vi "Terminal-Core-InitializeNotifiers.vi"(0 "comand (Initialize)":enum16{"UnInitialize", "Initialize"}(ring), 11 "error in (no error)":errorcluster caption="错误输入（无错误）") -> (1 "LoadingUnitNRef":refnum<notifier>, 2 "LubricateUnitNRef":refnum<notifier>, 3 "DeviceLubricateUnitNRef":refnum<notifier>, 4 "ModbusNReqRef":refnum<notifier>, 6 "ModbusNResRef":refnum<notifier>, 8 "DriverSystemNRef":refnum<notifier>, 10 "GearSystemNRef":refnum<notifier>, 15 "error out":errorcluster caption="错误输出")   [LabVIEW 2014]
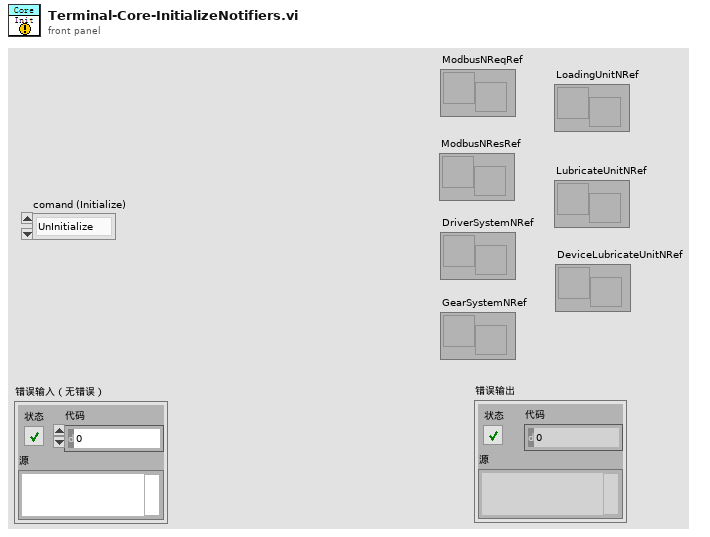
[diagram p1: front panel]
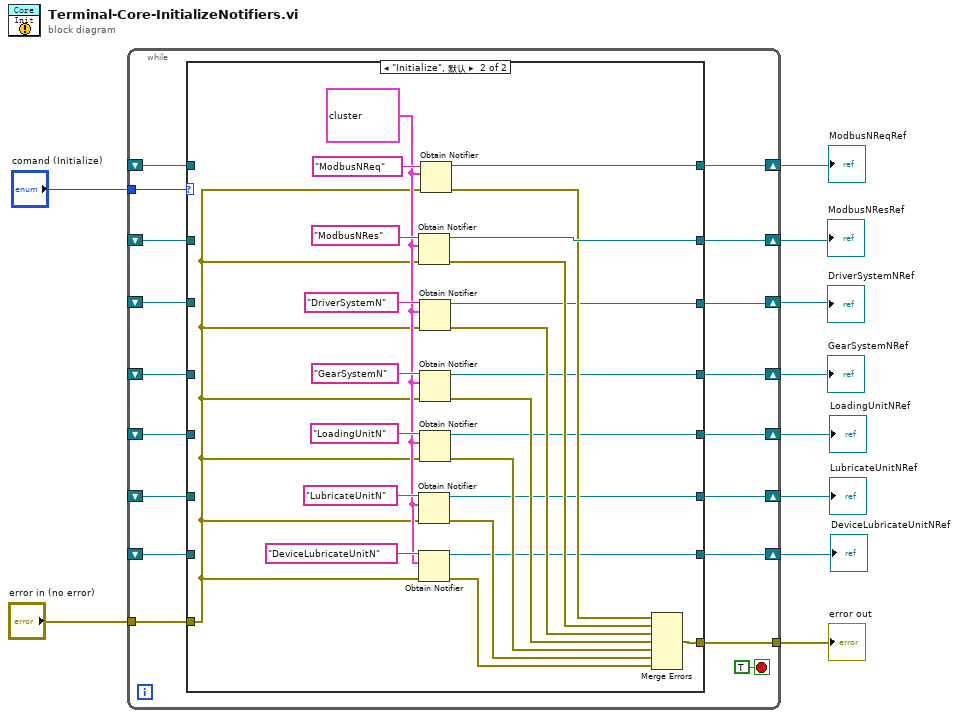
[diagram p0: block diagram]
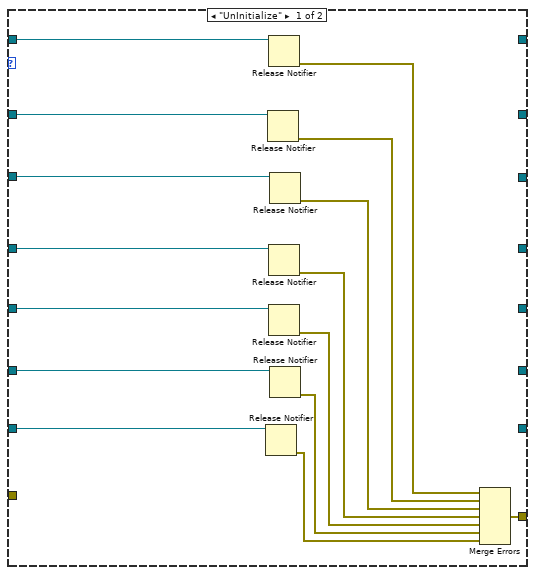
[diagram p2: hidden frame]
diagram:
  n1 = while {
    tunnel: "comand (Initialize)" -> [w27]
    tunnel: "error in (no error)" -> [w26]
    shift-right: [w25] -> w8
    shift-left: _ -> [w24]
    tunnel: [w23] -> w7
    shift-right: [w22] -> w6
    shift-left: _ -> [w21]
    shift-right: [w20] -> w5
    shift-left: _ -> [w19]
    shift-right: [w18] -> w4
    shift-left: _ -> [w14]
    shift-right: [w17] -> w3
    shift-left: _ -> [w13]
    shift-right: [w16] -> w2
    shift-left: _ -> [w12]
    shift-right: [w15] -> w1
    shift-left: _ -> [w11]
    stop <- TRUE stop-if-true
    n2 = case shown="\"Initialize\", 默认" w27 {
      tunnel: w26 -> [_ w52]
      tunnel: [_ w66] -> w25
      tunnel: w24 -> [w43 _]
      tunnel: [w40 w62] -> w23
      tunnel: [_ w64] -> w22
      tunnel: w21 -> [w42 _]
      tunnel: [_ w58] -> w20
      tunnel: w19 -> [w38 _]
      tunnel: [_ w47] -> w18
      tunnel: [_ w46] -> w17
      tunnel: [_ w45] -> w16
      tunnel: [_ w44] -> w15
      tunnel: w14 -> [w36 _]
      tunnel: w13 -> [w35 _]
      tunnel: w12 -> [w34 _]
      tunnel: w11 -> [w33 _]
      frame "UnInitialize" {
        n3 = Release Notifier(notifier=w33) -> (error out=w29:errorcluster)  [unwired: 2 in, 2 out]
        n4 = Release Notifier(notifier=w43) -> (error out=w39:errorcluster)  [unwired: 2 in, 2 out]
        n5 = Release Notifier(notifier=w42) -> (error out=w41:errorcluster)  [unwired: 2 in, 2 out]
        n6 = Release Notifier(notifier=w36) -> (error out=w32:errorcluster)  [unwired: 2 in, 2 out]
        n7 = Release Notifier(notifier=w35) -> (error out=w31:errorcluster)  [unwired: 2 in, 2 out]
        n8 = Release Notifier(notifier=w38) -> (error out=w37:errorcluster)  [unwired: 2 in, 2 out]
        n9 = Release Notifier(notifier=w34) -> (error out=w30:errorcluster)  [unwired: 2 in, 2 out]
        n10 = Merge Errors(w41, w39, w37, w32, w31, w30, w29) -> (w40:errorcluster)
      }
      frame "Initialize", Default {
        w53 = cluster{"Data":variant, "State":string} {"Data"=variant, "State"=""}
        n11 = Obtain Notifier(name (unnamed)="ModbusNRes" ("名称（未命名）"), notification data type=w53, error in (no error)=w52) -> (notifier out=w66:refnum<notifier>, error out=w61:errorcluster)  [unwired: 1 in, 1 out]
        n12 = Obtain Notifier(name (unnamed)="LubricateUnitN" ("名称（未命名）"), notification data type=w53, error in (no error)=w52) -> (notifier out=w45:refnum<notifier>, error out=w50:errorcluster)  [unwired: 1 in, 1 out]
        n13 = Obtain Notifier(name (unnamed)="DeviceLubricateUnitN" ("名称（未命名）"), notification data type=w53, error in (no error)=w52) -> (notifier out=w44:refnum<notifier>, error out=w51:errorcluster)  [unwired: 1 in, 1 out]
        n14 = Obtain Notifier(name (unnamed)="DriverSystemN" ("名称（未命名）"), notification data type=w53, error in (no error)=w52) -> (notifier out=w58:refnum<notifier>, error out=w60:errorcluster)  [unwired: 1 in, 1 out]
        n15 = Obtain Notifier(name (unnamed)="GearSystemN" ("名称（未命名）"), notification data type=w53, error in (no error)=w52) -> (notifier out=w47:refnum<notifier>, error out=w48:errorcluster)  [unwired: 1 in, 1 out]
        n16 = Obtain Notifier(name (unnamed)="LoadingUnitN" ("名称（未命名）"), notification data type=w53, error in (no error)=w52) -> (notifier out=w46:refnum<notifier>, error out=w49:errorcluster)  [unwired: 1 in, 1 out]
        n17 = Obtain Notifier(name (unnamed)="ModbusNReq" ("名称（未命名）"), notification data type=w53, error in (no error)=w52) -> (notifier out=w64:refnum<notifier>, error out=w63:errorcluster)  [unwired: 1 in, 1 out]
        n18 = Merge Errors(w63, w61, w60, w48, w49, w50, w51) -> (w62:errorcluster)
      }
    }
  }
  "error out" <- w7
  "ModbusNResRef" <- w8
  "ModbusNReqRef" <- w6
  "DriverSystemNRef" <- w5
  "GearSystemNRef" <- w4
  "LoadingUnitNRef" <- w3
  "LubricateUnitNRef" <- w2
  "DeviceLubricateUnitNRef" <- w1
